vi "ConnectDAQmx.vi"(8 "error in":errorcluster, 9 "Command":string, 10 "ON/OFF":bool, 11 "Control in":refnum<class "Control-Server.lvclass">) -> (0 "error out":errorcluster, 3 "Control out":refnum<class "Control-Server.lvclass">)   [LabVIEW 2020, in "Control-Server.lvclass"]
uses:
  Control-Server.lvclass
  dependecies/ControlsVIs/Clusters-def/Message types.ctl
  DAQmxTasks/DAQmxTaskContainer_General/DAQmxTaksContainer_General.lvclass
  C:/dev/TRANCON/Classes/GeneralFunctionality/GeneralFunctionality.lvclass
  Message/Message.lvclass
  GeneralFunctionality/GeneralFunctionality.lvclass
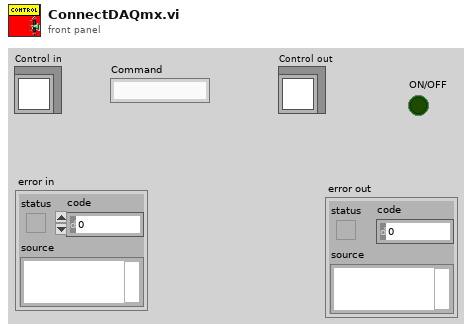
[diagram p1: front panel]
types:
  T1 = typedef "Message types.ctl" = string
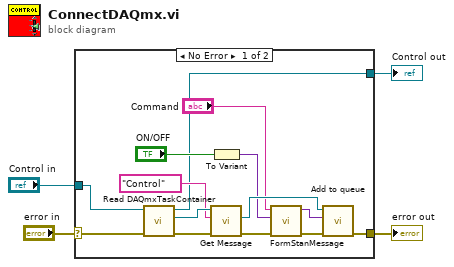
[diagram p0: block diagram]
diagram:
  n1 = case shown="No Error" "error in" {
    selector: "error in" -> [w12 w20]
    tunnel: "Control in" -> [w18 w19]
    tunnel: [w13 w19] -> w3
    tunnel: [w11 w20] -> w2
    frame No Error {
      n2 = call-dynamic "Read DAQmxTaskContainer.vi"("error in (no error)"=w12, "Control in"=w18) -> ("error out"=w17:errorcluster, "DAQmxTaksContainer_General.lvclass"=w16:refnum<class "DAQmxTaksContainer_General.lvclass">, "Control out"=w13:refnum<class "Control-Server.lvclass">)  [unwired: 7 in]
      n3 = call "Get Message.vi"("error in (no error)"=w17, "Message type"=T1 "Control", "GeneralFunctionality en entrée"=w16) -> ("error out"=w9:errorcluster, "Message.lvclass"=w10:refnum<class "Message.lvclass">)  [unwired: 6 in, 1 out]
      n4 = To Variant(anything="ON/OFF") -> (Variant=w7:variant)
      n5 = call "FormStanMessage.vi"("error in"=w9, "data"=w7, "Command"="Command") -> ("error out"=w8:errorcluster, "message"=w6:variant)  [unwired: 7 in]
      n6 = call "Add to queue.vi"("error in (no error)"=w8, "Data"=w6, "Message in"=w10) -> ("error out"=w11:errorcluster)  [unwired: 7 in, 1 out]
    }
    frame Error {
    }
  }
  "Control out" <- w3
  "error out" <- w2
